vi "call_from_memory.vi"(2 "Column":i32, 3 "Row":i32, 4 "Memory":T1) -> (0 "Array Element":u8, 1 "Memory Out":T1)   [LabVIEW 2009]
uses:
  behaviors/occupancy grid memory typedef.ctl
  <vilib>/rvi/DataTransferAndStorage/Container/XNode/niFpgaContainer.xnode
  <vilib>/rvi/DataTransferAndStorage/Container/Common/niFpgaContainerExecOnDevCompGetState.vi
  <vilib>/rvi/DataTransferAndStorage/Container/Common/niFpgaContainerMetaDataKey.ctl
  <vilib>/rvi/Memory/Memory_Emulation/nirvimemoryEmulationManagerCache_GetValue.vi
  <vilib>/rvi/Memory/Memory_Emulation/nirvimemoryEmulationManagerCache_InsertValue.vi
  <vilib>/rvi/FIFO/Fifo_Resource/nirvififoUniquifyingName.vi
  <vilib>/Utility/error.llb/Clear Errors.vi
  <vilib>/rvi/Memory/Memory_Emulation/nirvimemoryEmulationManagerCache_SetValue.vi
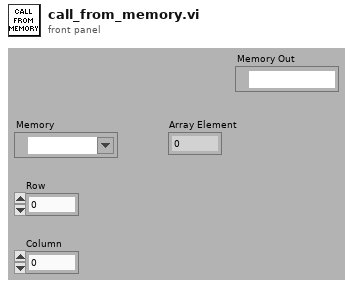
[diagram p1: front panel]
types:
  T1 = typedef "occupancy grid memory typedef.ctl" = refnum<k21>
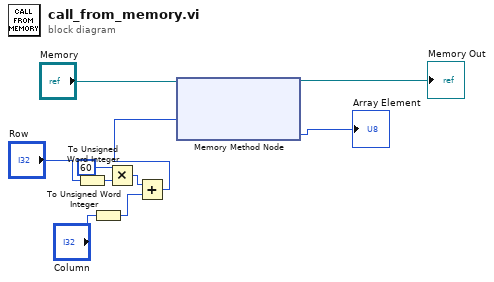
[diagram p0: block diagram]
diagram:
  n1 = To Unsigned Word Integer(number="Row") -> (unsigned 16bit integer=w4:u16)
  n2 = To Unsigned Word Integer(number="Column") -> (unsigned 16bit integer=w7:u16)
  n3 = Multiply(x=u16 60, y=w4) -> (x*y=w6:u16)
  n4 = Add(x=w6, y=w7) -> (x+y=w8:u16)
  n5 = xnode ("Memory Method Node")("Address"=w8, "Memory In"="Memory") -> ("Data"=→"Array Element":i8, "Memory Out"=→"Memory Out":T1)
